vi "Rotation stage shg.vi"() -> ()   [LabVIEW 2020]
doc: "Shows how to move a motor to an absolute position."
uses:
  <vilib>/DAQmx/read.llb/DAQmx Read (Counter 1D U32 1Chan NSamp).vi
  <vilib>/DAQmx/create/channels.llb/DAQmx Create Channel (CI-Period).vi
  <vilib>/DAQmx/configure/timing.llb/DAQmx Timing (Implicit).vi
  <vilib>/DAQmx/create/channels.llb/DAQmx Create Channel (CO-Pulse Generation-Frequency).vi
  <vilib>/DAQmx/miscellaneous.llb/DAQmx Fill In Error Info.vi
  <resource>/objmgr/daqmx.rc
  <vilib>/Analysis/NI_AALBase.lvlib
panel:
  in  "samples per loop":i32=1
  out "count":u32[](array[numeric])
  in  "stop":bool
  out "Waveform Chart":u32[](graph)
  out "Waveform Chart 2":dynamicdata(graph)
  out "Ref. Channel":dbl(graph)
  in  "samples per loop ref":i32=1
  out "Numeric Indicator":dbl
  out "mean":dbl(graph)
  in  "dwell time (ms)":dbl=1.0 format="%.6f"
  in  "Photon Input (PFI)":tag="/Dev1/PFI0"
  in  "Rotation Angle (Degrees)":dbl=100.0 min=0.0
  in  "MG17Motor":refnum<k7>(container)
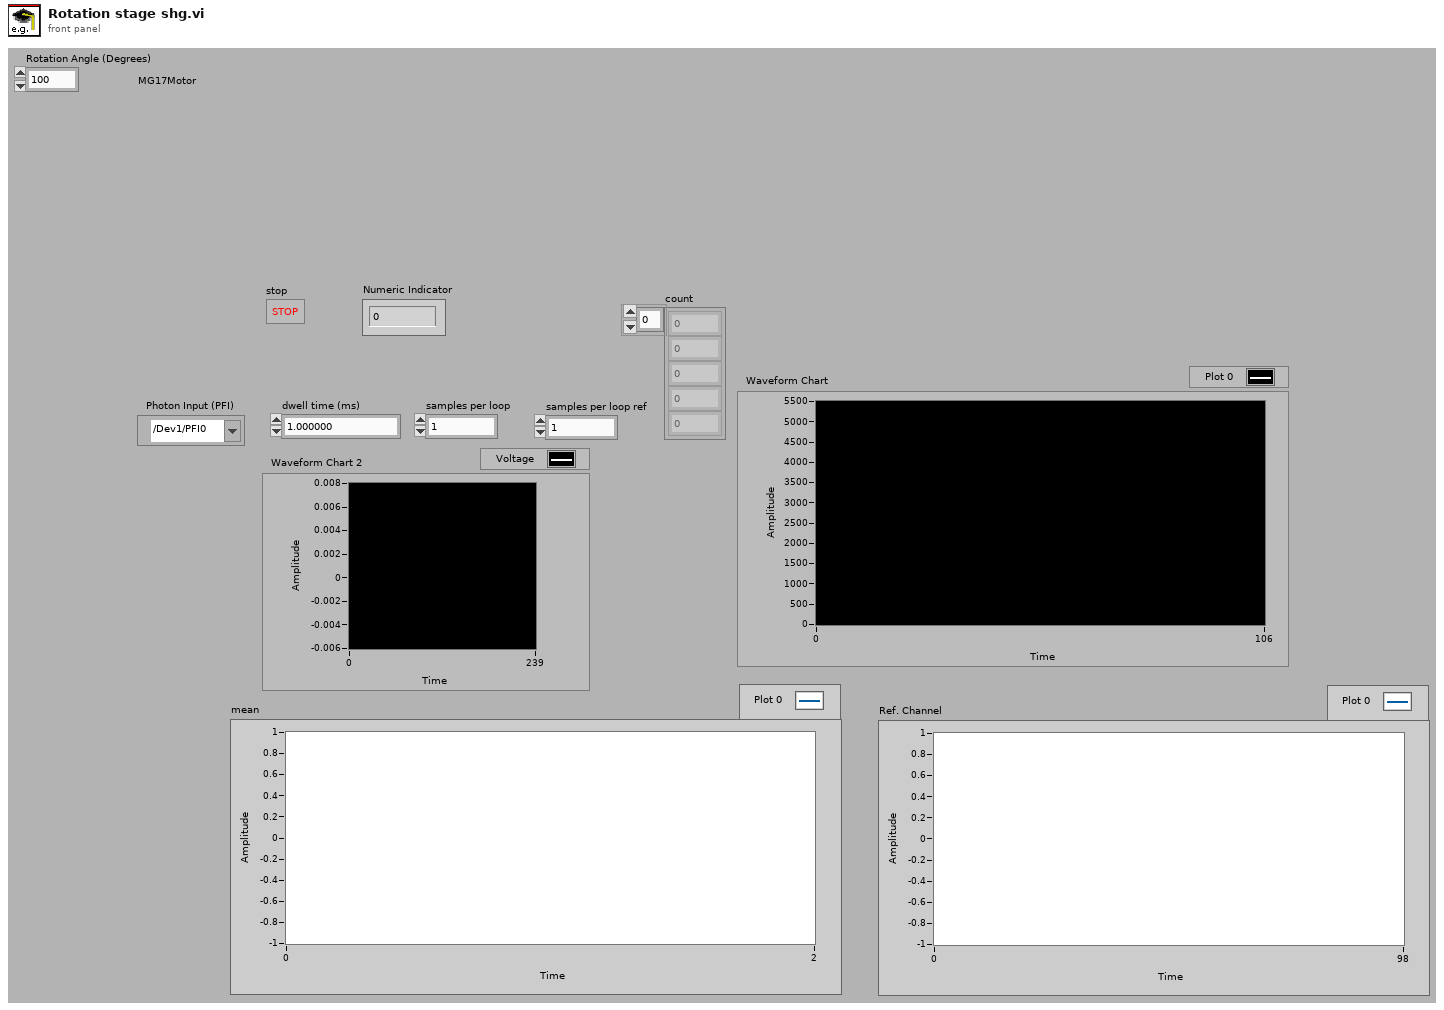
[diagram p1: front panel]
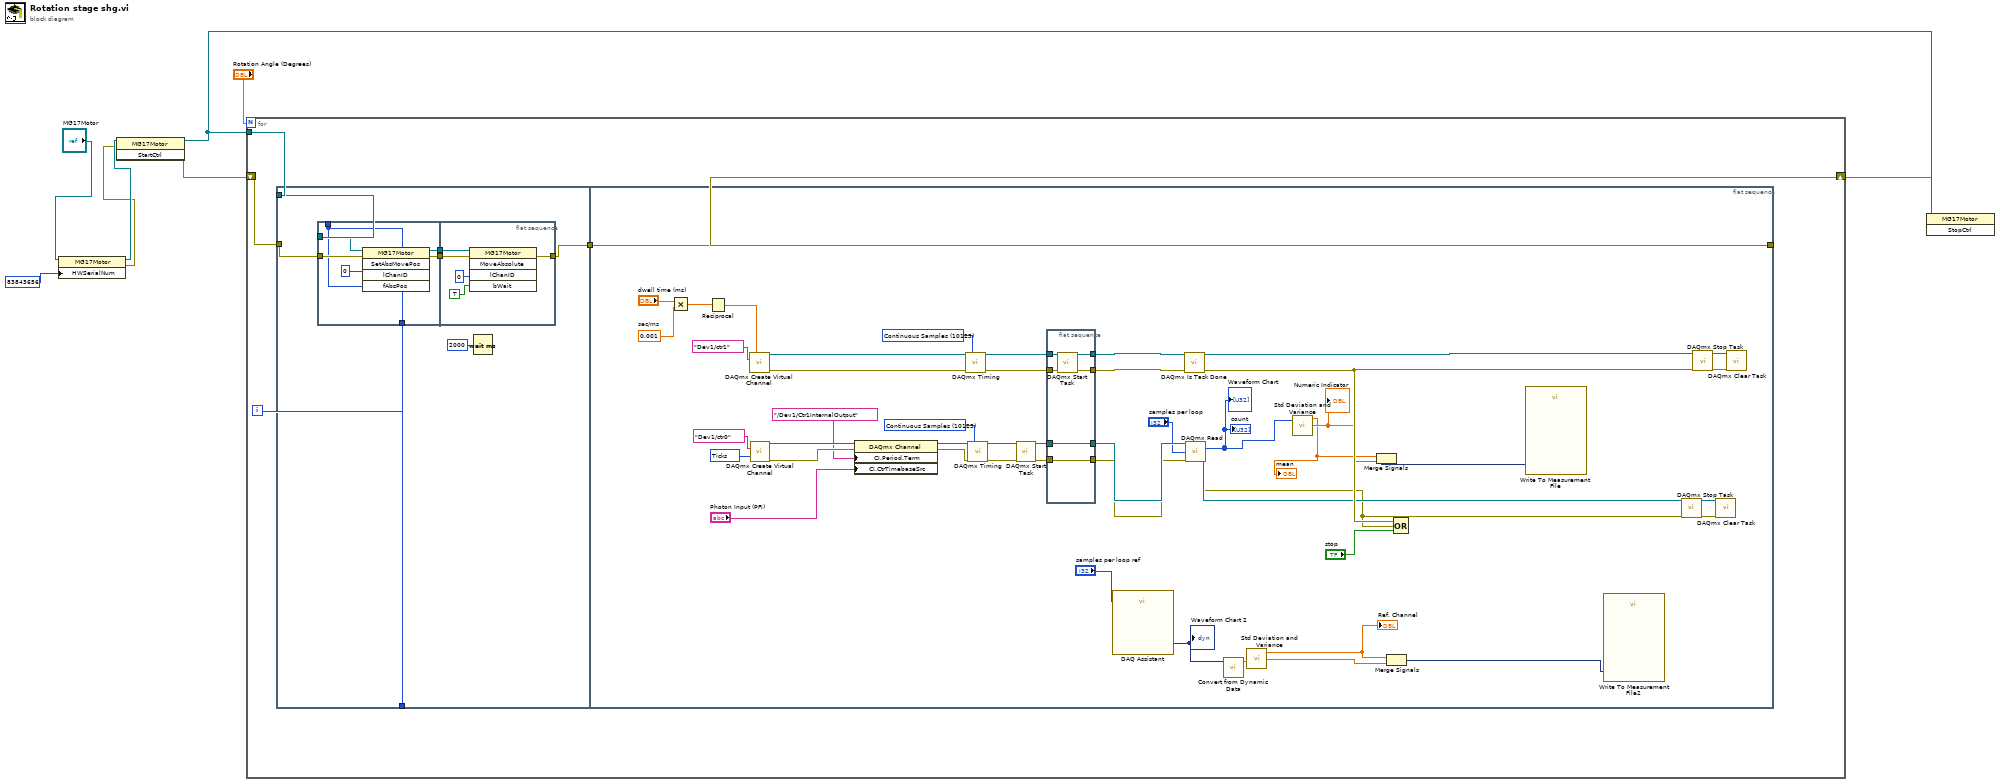
[diagram p0: block diagram]
diagram:
  n1 = property class="MG17Motor"(reference="MG17Motor", "HWSerialNum"=83843656) -> (reference out=w4:refnum<k7>, error out=w3:errorcluster)  [unwired: 1 in]
  n2 = invoke class="MG17Motor" method="StartCtrl"(reference=w4, error in=w3) -> (reference out=w8:refnum<k7>, error out=w7:errorcluster)  [unwired: 1 in, 1 out]
  n3 = for {
    N: "Rotation Angle (Degrees)" -> [_]
    tunnel: w8 -> [w13]
    shift-right: [w11] -> w6
    shift-left: w7 -> [w12]
    i -> [w9]
    n4 = flat-sequence {
      tunnel: w13 -> [w18]
      tunnel: w12 -> [w16]
      tunnel: [w15] -> w10
      tunnel: w9 -> [w17]
      tunnel: [w79] -> w11
      tunnel: w10 -> [w79]
      frame #0 {
        n5 = flat-sequence {
          tunnel: [w21] -> _
          tunnel: w16 -> [w25]
          tunnel: w18 -> [w24]
          tunnel: [w23] -> w20
          tunnel: [w22] -> w19
          tunnel: w17 -> [w21]
          tunnel: w20 -> [w29]
          tunnel: w19 -> [w28]
          tunnel: [w27] -> w15
          frame #0 {
            n6 = invoke class="MG17Motor" method="SetAbsMovePos"(reference=w24, error in=w25, "lChanID"=0, "fAbsPos"=w21) -> (reference out=w22:refnum<k7>, error out=w23:errorcluster)  [unwired: 1 in, 3 out]
          }
          frame #1 {
            n7 = invoke class="MG17Motor" method="MoveAbsolute"(reference=w28, error in=w29, "lChanID"=0, "bWait"=TRUE) -> (error out=w27:errorcluster)  [unwired: 1 in, 4 out]
          }
        }
        n8 = Wait (ms)(milliseconds to wait=u32 2000) -> ()  [unwired: 1 out]
      }
      frame #1 {
        w50 = 0.001  # sec/ms
        w60 = 10304 items=["Seconds"=10364, "Ticks"=10304, "From Custom Scale"=10065] ("units")
        w61 = 10123 items=["Finite Samples"=10178, "Continuous Samples"=10123, "Hardware Timed Single Point"=12522] ("sample mode")
        w62 = 10123 items=["Finite Samples"=10178, "Continuous Samples"=10123, "Hardware Timed Single Point"=12522] ("sample mode")
        n9 = Multiply(x="dwell time (ms)", y=w50) -> (x*y=w49:dbl)
        n10 = Reciprocal(x=w49) -> (1/x=w48:dbl)
        n11 = call-poly <vilib>:"DAQmx Create Virtual Channel.vi"("frequency"=w48, "counter"=tag "Dev1/ctr1") -> ("task out"=w77:refnum<k21>, "error out"=w78:errorcluster)  [unwired: 12 in]
        n12 = call-poly <vilib>:"DAQmx Create Virtual Channel.vi"("counter"=tag "Dev1/ctr0", "units"=w60) -> ("task out"=w57:refnum<k21>, "error out"=w56:errorcluster)  [unwired: 12 in]
        n13 = property class="DAQmx Channel"(reference=w57, error in=w56, "CI.Period.Term"=tag "/Dev1/Ctr1InternalOutput", "CI.CtrTimebaseSrc"="Photon Input (PFI)") -> (reference out=w55:refnum<k21>, error out=w54:errorcluster)
        n14 = call-poly <vilib>:"DAQmx Timing.vi"("task/channels in"=w77, "sample mode"=w62, "error in"=w78) -> ("task out"=w76:refnum<k21>, "error out"=w75:errorcluster)  [unwired: 11 in]
        n15 = call-poly <vilib>:"DAQmx Timing.vi"("task/channels in"=w55, "sample mode"=w61, "error in"=w54) -> ("task out"=w68:refnum<k21>, "error out"=w67:errorcluster)  [unwired: 11 in]
        n16 = call <vilib>:"DAQmx Start Task.vi"("task/channels in"=w68, "error in"=w67) -> ("task out"=w46:refnum<k21>, "error out"=w44:errorcluster)  [unwired: 12 in]
        n17 = flat-sequence {
          tunnel: w76 -> [w85]
          tunnel: w75 -> [w84]
          tunnel: [w83] -> w74
          tunnel: [w82] -> w73
          tunnel: [w81] -> w47
          tunnel: w46 -> [w81]
          tunnel: [w80] -> w45
          tunnel: w44 -> [w80]
          frame #0 {
            n18 = call <vilib>:"DAQmx Start Task.vi"("task/channels in"=w85, "error in"=w84) -> ("task out"=w82:refnum<k21>, "error out"=w83:errorcluster)  [unwired: 12 in]
          }
        }
        n19 = call "DAQ Assistant"("number of samples"="samples per loop ref") -> ("data"=w42:dynamicdata)  [unwired: 16 in, 2 out]
        "Waveform Chart 2" <- w42
        n20 = call <vilib>:"DAQmx Is Task Done.vi"("task/channels in"=w73, "error in"=w74) -> ("task out"=w71:refnum<k21>, "error out"=w72:errorcluster)  [unwired: 11 in, 1 out]
        n21 = call-poly <vilib>:"DAQmx Read.vi"("task/channels in"=w47, "number of samples per channel"="samples per loop", "error in"=w45) -> ("task out"=w66:refnum<k21>, "data"=w34:u32[], "error out"=w65:errorcluster)  [unwired: 10 in]
        "count" <- w34
        "Waveform Chart" <- w34
        n22 = call "Convert from Dynamic Data"("Dynamic Data Type"=w42) -> ("Array"=w41:dbl[])  [unwired: 3 in]
        n23 = call <vilib>:"Std Deviation and Variance.vi"("X"=w41) -> ("mean"=w40:dbl, "standard deviation"=w39:dbl)  [unwired: 1 in, 1 out]
        "Ref. Channel" <- w40
        n24 = call <vilib>:"Std Deviation and Variance.vi"("X"=w34) -> ("mean"=w32:dbl, "standard deviation"=w33:dbl)  [unwired: 1 in, 1 out]
        "Numeric Indicator" <- w33
        "mean" <- w32
        n25 = Merge Signals(w32, w33) -> (w37:dynamicdata)
        n26 = Merge Signals(w40, w39) -> (w43:dynamicdata)
        n27 = Compound Arithmetic op=OR(w72, w65, "stop") -> ()  [unwired: 1 out]
        n28 = call "Write To Measurement File"("Signals"=w37) -> ()  [unwired: 16 in, 3 out]
        n29 = call "Write To Measurement File2"("Signals"=w43) -> ()  [unwired: 16 in, 3 out]
        n30 = call <vilib>:"DAQmx Stop Task.vi"("task/channels in"=w66, "error in"=w65) -> ("task out"=w63:refnum<k21>, "error out"=w64:errorcluster)  [unwired: 12 in]
        n31 = call <vilib>:"DAQmx Stop Task.vi"("task/channels in"=w71, "error in"=w72) -> ("task out"=w70:refnum<k21>, "error out"=w69:errorcluster)  [unwired: 12 in]
        n32 = call <vilib>:"DAQmx Clear Task.vi"("task in"=w63, "error in"=w64) -> ()  [unwired: 13 in, 1 out]
        n33 = call <vilib>:"DAQmx Clear Task.vi"("task in"=w70, "error in"=w69) -> ()  [unwired: 13 in, 1 out]
      }
    }
  }
  n34 = invoke class="MG17Motor" method="StopCtrl"(reference=w8, error in=w6) -> ()  [unwired: 1 in, 3 out]
